vi "OAT Set Timebase Plot Property.vi"(5 "Y axis graph Ref":refnum<vi>, 7 "X axis graph Ref":refnum<vi>, 8 "orbit color settings":T1={"tach point color"=16711680, "orbit plot color"=16777226}, 10 "Y axis in":cluster{"X":dbl[], "Y":dbl[]}[](array[cluster]) {"Y" format="%.2f"; "X" format="%.2f"}, 11 "x axis in":cluster{"X":dbl[], "Y":dbl[]}[](array[cluster]) {"Y" format="%.2f"; "X" format="%.2f"}) -> (2 "Y axis Plot":cluster{"X":dbl[], "Y":dbl[]}[](array[cluster]) {"Y" format="%.2f"; "X" format="%.2f"}, 3 "X axis Plot":cluster{"X":dbl[], "Y":dbl[]}[](array[cluster]) {"Y" format="%.2f"; "X" format="%.2f"})   [LabVIEW 2017]
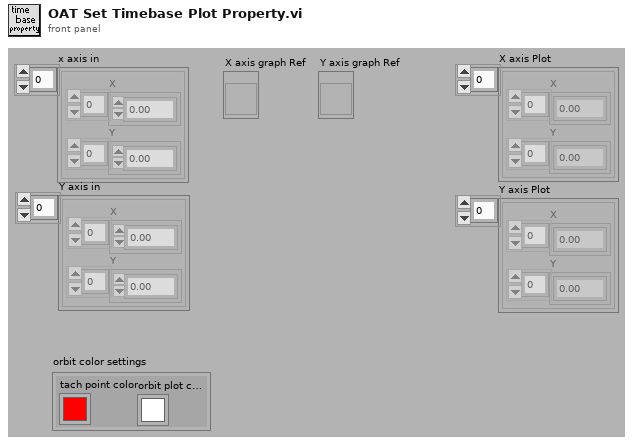
[diagram p1: front panel]
types:
  T1 = cluster{"tach point color":u32, "orbit plot color":u32}
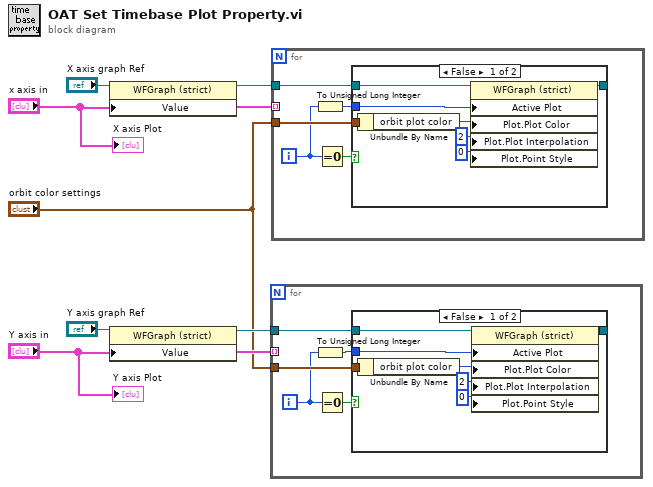
[diagram p0: block diagram]
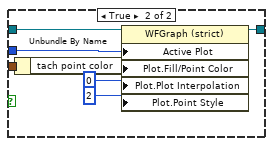
[diagram p2: hidden frame]
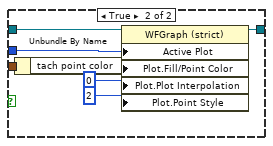
[diagram p3: hidden frame]
diagram:
  n1 = property class="WFGraph (strict)"(reference="X axis graph Ref", "Value"="x axis in") -> (reference out=w5:refnum<vi>)  [unwired: 1 in, 1 out]
  n2 = property class="WFGraph (strict)"(reference="Y axis graph Ref", "Value"="Y axis in") -> (reference out=w2:refnum<vi>)  [unwired: 1 in, 1 out]
  n3 = for {
    tunnel: "Y axis in" -> [_] mode=indexing
    tunnel: w2 -> [w10]
    tunnel: "orbit color settings" -> [w9]
    i -> [w8]
    n4 = To Unsigned Long Integer(number=w8) -> (unsigned 32bit integer=w11:u32)
    n5 = Equal To 0?(x=w8) -> (x = 0?=w12:bool)
    n6 = case shown="False" w12 {
      tunnel: w9 -> [w19 w26]
      tunnel: w10 -> [w18 w25]
      tunnel: w11 -> [w17 w24]
      tunnel: [w13 w20] -> _
      frame False {
        n7 = Unbundle By Name(w19) -> ("orbit plot color"=w16:u32)
        n8 = property class="WFGraph (strict)"(reference=w18, "Active Plot"=w17, "Plot.Plot Color"=w16, "Plot.Plot Interpolation"=u8 2, "Plot.Point Style"=u8 0) -> (reference out=w13:refnum<vi>)  [unwired: 1 in, 1 out]
      }
      frame True {
        n9 = Unbundle By Name(w26) -> ("tach point color"=w23:u32)
        n10 = property class="WFGraph (strict)"(reference=w25, "Active Plot"=w24, "Plot.Fill/Point Color"=w23, "Plot.Plot Interpolation"=u8 0 ("Plot.Point Style"), "Plot.Point Style"=u8 2 ("Plot.Plot Interpolation")) -> (reference out=w20:refnum<vi>)  [unwired: 1 in, 1 out]
      }
    }
  }
  n11 = for {
    tunnel: "x axis in" -> [_] mode=indexing
    tunnel: w5 -> [w29]
    tunnel: "orbit color settings" -> [w28]
    i -> [w27]
    n12 = To Unsigned Long Integer(number=w27) -> (unsigned 32bit integer=w30:u32)
    n13 = Equal To 0?(x=w27) -> (x = 0?=w31:bool)
    n14 = case shown="False" w31 {
      tunnel: w28 -> [w38 w45]
      tunnel: w29 -> [w37 w44]
      tunnel: w30 -> [w36 w43]
      tunnel: [w32 w39] -> _
      frame False {
        n15 = Unbundle By Name(w38) -> ("orbit plot color"=w35:u32)
        n16 = property class="WFGraph (strict)"(reference=w37, "Active Plot"=w36, "Plot.Plot Color"=w35, "Plot.Plot Interpolation"=u8 2, "Plot.Point Style"=u8 0) -> (reference out=w32:refnum<vi>)  [unwired: 1 in, 1 out]
      }
      frame True {
        n17 = Unbundle By Name(w45) -> ("tach point color"=w42:u32)
        n18 = property class="WFGraph (strict)"(reference=w44, "Active Plot"=w43, "Plot.Fill/Point Color"=w42, "Plot.Plot Interpolation"=u8 0 ("Plot.Point Style"), "Plot.Point Style"=u8 2 ("Plot.Plot Interpolation")) -> (reference out=w39:refnum<vi>)  [unwired: 1 in, 1 out]
      }
    }
  }
  "X axis Plot" <- "x axis in"
  "Y axis Plot" <- "Y axis in"
